vi "Filter Expected Execution Errors.vi"(8 "error in":errorcluster, 11 "N":i32) -> (0 "error out":errorcluster)   [LabVIEW 2020, in "Get GPU Device Information.lvlib"]
uses:
  Get GPU Device Information.lvlib
  <vilib>/addons/lvgpu/lvcuda/LVCUDA Error Code.ctl
  <vilib>/addons/lvgpu/lvcuda.lvlib
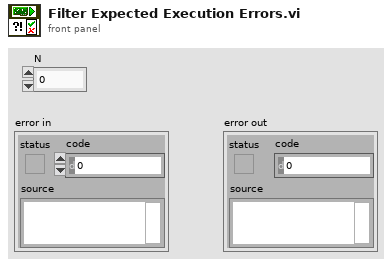
[diagram p1: front panel]
types:
  T1 = typedef "lvcuda.lvlib/LVCUDA Error Code.ctl" = i32
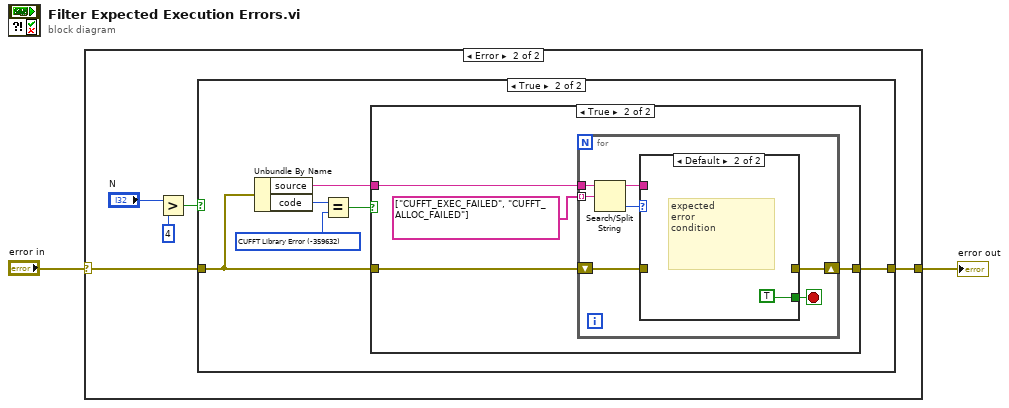
[diagram p0: block diagram]
diagram:
  n1 = case shown="Error" "error in" {
    selector: "error in" -> [w3 w8]
    tunnel: [w3 w7] -> w2
    frame No Error {
    }
    frame Error {
      n2 = Greater?(x="N", y=4) -> (0:w6:bool)
      n3 = case shown="True" w6 {
        tunnel: w8 -> [w9 w15]
        tunnel: [w9 w14] -> w7
        frame False {
          # "Expected failures codes produced in the first few iterations of the test are treated as errors. The FFTs performed initially are very small and should pass on any GPU device."
        }
        frame True {
          w10 = T1 -359632 items=["No Error"=0, "Array Dimension Mismatch"=-359610, "Unlock Data Mismatch"=-359620, "CUBLAS Library Error"=-359630, "CUDA Toolkit Library Error"=-359631, "CUFFT Library Error"=-359632, "CUDA Driver Library Error"=-359633] ("LVCUFFT Error Code")
          n4 = Unbundle By Name(w15) -> ("source"=w12:string, "code"=w11:i32)
          n5 = Equal?(x=w11, y=w10) -> (x = y?=w13:bool)
          n6 = case shown="True" w13 {
            tunnel: w15 -> [w16 w19]
            tunnel: [w16 w18] -> w14
            tunnel: w12 -> [_ w20]
            frame False {
            }
            frame True {
              n7 = for {
                tunnel: w20 -> [w26]
                tunnel: string[] ["CUFFT_EXEC_FAILED", "CUFFT_ALLOC_FAILED"] -> [w22] mode=indexing
                shift-right: [w24] -> w18
                shift-left: w19 -> [w25]
                stop <- w21 stop-if-true
                n8 = Search/Split String(string=w26, search string/char (-)=w22) -> (substring before match=w23:string, offset of match=w27:i32)  [unwired: 1 in, 1 out]
                n9 = case shown="Default" w27 {
                  tunnel: w25 -> [w28 _]
                  tunnel: [w28 _] -> w24
                  tunnel: w23 -> [_ _]
                  tunnel: [_ TRUE] -> w21
                  frame -1 {
                  }
                  frame Default {
                    # "expected\nerror\ncondition"
                  }
                }
              }
            }
          }
        }
      }
    }
  }
  "error out" <- w2
